vi "setScale.vi"(8 "Error In":errorcluster, 9 "upperBound":dbl, 10 "lowerBound":dbl, 11 "QwtAbstractScale In":refnum<class "QwtAbstractScale.lvclass">) -> (0 "Error Out":errorcluster, 3 "QwtAbstractScale Out":refnum<class "QwtAbstractScale.lvclass">)   [LabVIEW 2014, in "QwtAbstractScale.lvclass"]
doc: "LabVIEW-specific documentation is not yet available. See <b>http://qwt.sourceforge.net/class_qwt_abstract_scale.html#setScale</b>"
uses:
  QwtAbstractScale.lvclass
  LQ Core/LQIdentity/LQIdentity.lvclass/LQIdentity.ctl
  LQ Core/LQ Core.lvlib
  LQ Core/LQIdentity/LQIdentity.lvclass
panel:
  # "Copyright (c) 2016 Sze Howe Koh\n\nThis Source Code Form is subject to the terms of the Mozilla Public\nLicense, v. 2.0. If a copy of the MPL was not distributed with this\nfile, You can obtain one at http://mozilla.org/MPL/2.0/."
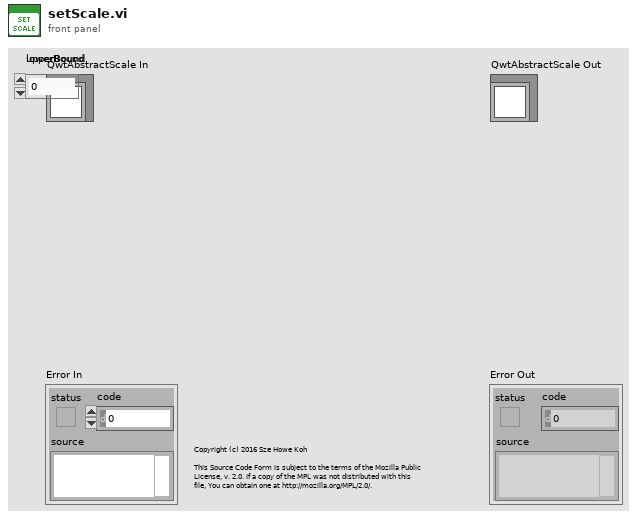
[diagram p1: front panel]
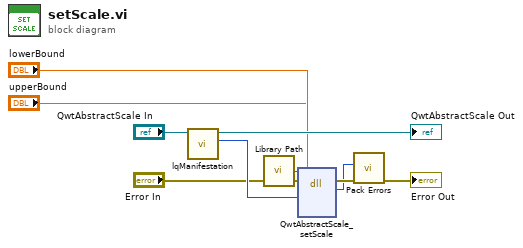
[diagram p0: block diagram]
diagram:
  n1 = call "lqManifestation.vi"("LQIdentity in"="QwtAbstractScale In") -> ("Manifestation"=w7:u64, "LQIdentity out"=→"QwtAbstractScale Out":refnum<class "QwtAbstractScale.lvclass">)  [unwired: 9 in]
  n2 = call "Library Path.vi"() -> ("Library Path"=w8:path)
  n3 = dll-call lib="?" fn="QwtAbstractScale_setScale"(path in=w8, error in="Error In", "_instance"=w7, "lowerBound"="lowerBound", "upperBound"="upperBound") -> (error out=w5:errorcluster, w3:i32)  [unwired: 4 in, 1 out]
  n4 = call "Pack Errors.vi"("Error In"=w5, "Error Code"=w3) -> ("Error Out"=→"Error Out":errorcluster)  [unwired: 9 in]
